vi "Get Measurement Details.vi"(8 "error in":errorcluster, 11 "MeasurementPluginService in":refnum<class "Measurement Plugin Service.lvclass">) -> (0 "error out":errorcluster, 1 "Service Class":string, 2 "Measurement Details":T2, 3 "MeasurementPluginService out":refnum<class "Measurement Plugin Service.lvclass">, 4 "Measurement Annotations":T1[](array[typedef]))   [LabVIEW 2020, in "MeasurementLink Measurement Server.lvlib" / "Measurement Plugin Service.lvclass"]
uses:
  Measurement Plugin Service.lvclass
  Helpers/TypeDefs/Measurement Details.ctl
  Helpers/TypeDefs/Measurement Annotation.ctl
  MeasurementLink Measurement Server.lvlib
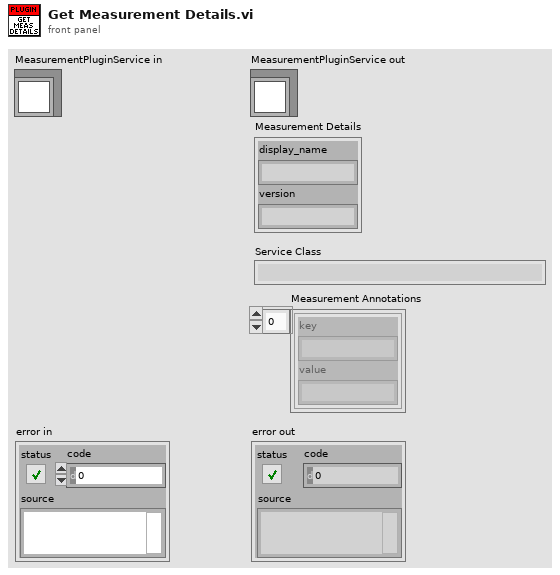
[diagram p1: front panel]
types:
  T1 = typedef "MeasurementLink Measurement Server.lvlib/Measurement Annotation.ctl" = cluster{"key":string, "value":string}
  T2 = typedef "MeasurementLink Measurement Server.lvlib/Measurement Details.ctl" = cluster{"display_name":string, "version":string}
  T3 = typedef "MeasurementLink Measurement Server.lvlib/Measurement Plugin Service.lvclass/Plugin Paths.ctl" = cluster{"Get Measurement Details VI Path":path, "Get Type Specializations VI Path":path, "Get UI Details VI Path":path, "Measurement Logic VI Path":path, "Measurement Configuration CTL Path":path, "Measurement Results CTL Path":path}
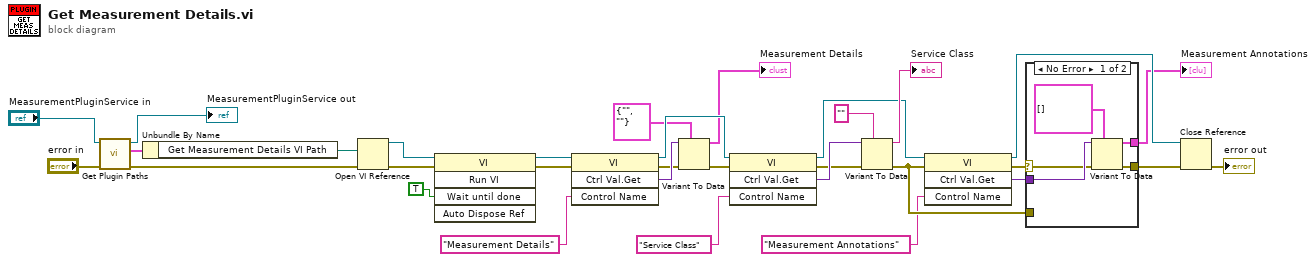
[diagram p0: block diagram]
diagram:
  n1 = call-dynamic "Get Plugin Paths.vi"("error in (no error)"="error in", "MeasurementPluginService in"="MeasurementPluginService in") -> ("error out"=w12:errorcluster, "Plugin Paths"=w29:T3, "MeasurementPluginService out"=→"MeasurementPluginService out":refnum<class "Measurement Plugin Service.lvclass">)  [unwired: 7 in]
  n2 = Unbundle By Name(w29) -> ("Get Measurement Details VI Path"=w14:path)
  n3 = Open VI Reference(vi path=w14, error in (no error)=w12) -> (vi reference=w28:refnum<vi>, error out=w21:errorcluster)  [unwired: 4 in]
  n4 = invoke class="VI" method="Run VI"(reference=w28, error in=w21, "Wait until done"=TRUE ("Wait Until Done")) -> (reference out=w26:refnum<vi>, error out=w22:errorcluster)  [unwired: 2 in, 3 out]
  n5 = invoke class="VI" method="Ctrl Val.Get"(reference=w26, error in=w22, "Control Name"="Measurement Details") -> (reference out=w23:refnum<vi>, error out=w19:errorcluster, "Get Control Value Variant"=w20:variant)  [unwired: 1 in, 1 out]
  n6 = Variant To Data(error in=w19, type=T2 {"display_name"="", "version"=""} ("MeasurementDetails"), Variant=w20) -> (data=→"Measurement Details":T2, error out=w18:errorcluster)
  n7 = invoke class="VI" method="Ctrl Val.Get"(reference=w23, error in=w18, "Control Name"="Service Class") -> (reference out=w7:refnum<vi>, error out=w16:errorcluster, "Get Control Value Variant"=w17:variant)  [unwired: 1 in, 1 out]
  n8 = Variant To Data(error in=w16, type="", Variant=w17) -> (data=→"Service Class":string, error out=w5:errorcluster)
  n9 = invoke class="VI" method="Ctrl Val.Get"(reference=w7, error in=w5, "Control Name"="Measurement Annotations") -> (reference out=w6:refnum<vi>, error out=w2:errorcluster, "Get Control Value Variant"=w4:variant)  [unwired: 1 in, 1 out]
  n10 = case shown="No Error" w2 {
    selector: w2 -> [w34 _]
    tunnel: [w37 w38] -> w8
    tunnel: w4 -> [w36 _]
    tunnel: [w35 _] -> w1
    tunnel: w5 -> [_ w38]
    frame No Error {
      n11 = Variant To Data(error in=w34, type=T1[] [], Variant=w36) -> (data=w35:T1[], error out=w37:errorcluster)
    }
    frame Error {
    }
  }
  "Measurement Annotations" <- w1
  n12 = Close Reference(reference=w6, error in (no error)=w8) -> (error out=→"error out":errorcluster)
